vi "Configure Standard Waveform.vi"(5 "Start Phase (0)":dbl, 6 "DC Offset (0 V)":dbl, 7 "Frequency (100000 Hz)":dbl=100000.0, 8 "error in (no error)":errorcluster, 9 "Amplitude (0.5 V)":dbl=0.5, 10 "Waveform Function (0: Sine)":i32(ring) items=["Sine", "Square", "Pulse", "Ramp", "Noise", "DC", "Sinc", "Gaussian", "Lorentz", "Exponential Rise", "Exponential Decay", "Haversine", "Cardiac"], 11 "VISA resource name":refnum<visa-resource-name>) -> (0 "error out":errorcluster, 3 "VISA resource name out":refnum<visa-resource-name>)   [LabVIEW 2017, in "Scope.lvlib" / "Tektronix DPO MSO 2000 4000 Series.lvlib"]
doc: "Configures the parameters of the function generator that affect standard waveform generation.\n\n<B>Notes:</B>\n(1) This VI is available for MDO3000 Series only.\n\n(2) Requires the MDO3AFG option to be installed.\n\n(3) <B>Configure Output Impedance</B> VI must be used before this VI, so that saved setups are recalled with the proper load factor applied."
uses:
  Tektronix DPO MSO 2000 4000 Series.lvlib
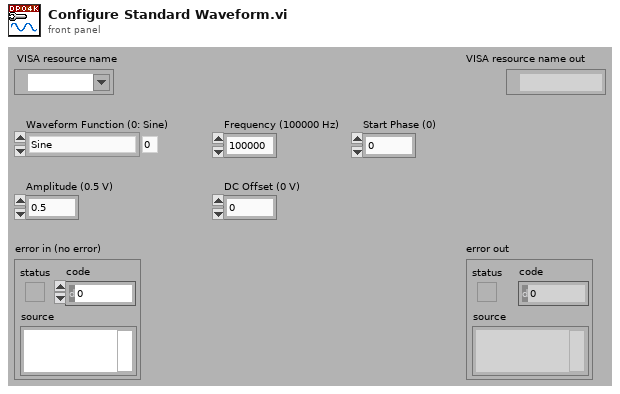
[diagram p1: front panel]
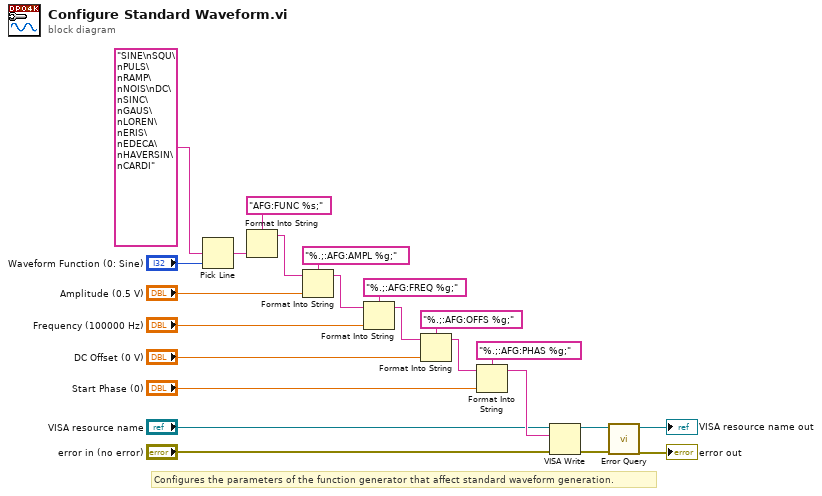
[diagram p0: block diagram]
diagram:
  # "Configures the parameters of the function generator that affect standard waveform generation."
  n1 = Pick Line(multi-line string="SINE\nSQU\nPULS\nRAMP\nNOIS\nDC\nSINC\nGAUS\nLOREN\nERIS\nEDECA\nHAVERSIN\nCARDI", line index="Waveform Function (0: Sine)") -> (output string=w2:string)  [unwired: 1 in]
  n2 = Format Into String(format string="AFG:FUNC %s;", w2) -> (resulting string=w1:string)  [unwired: 2 in, 1 out]
  n3 = Format Into String(format string="%.;:AFG:AMPL %g;", initial string=w1, "Amplitude (0.5 V)") -> (resulting string=w7:string)  [unwired: 1 in, 1 out]
  n4 = Format Into String(format string="%.;:AFG:FREQ %g;", initial string=w7, "Frequency (100000 Hz)") -> (resulting string=w6:string)  [unwired: 1 in, 1 out]
  n5 = Format Into String(format string="%.;:AFG:OFFS %g;", initial string=w6, "DC Offset (0 V)") -> (resulting string=w5:string)  [unwired: 1 in, 1 out]
  n6 = Format Into String(format string="%.;:AFG:PHAS %g;", initial string=w5, "Start Phase (0)") -> (resulting string=w14:string)  [unwired: 1 in, 1 out]
  n7 = VISA Write(VISA resource name="VISA resource name", write buffer=w14, error in (no error)="error in (no error)") -> (VISA resource name out=w12:refnum<visa-resource-name>, error out=w11:errorcluster)  [unwired: 1 out]
  n8 = call "Error Query.vi"("error in (no error)"=w11, "VISA resource name"=w12) -> ("error out"=→"error out":errorcluster, "VISA resource name out"=→"VISA resource name out":refnum<visa-resource-name>)  [unwired: 6 in, 2 out]
